vi "Register Event.vi"(4 "Get Last Broadcast Event (F)":bool, 6 "Event Handler":refnum<class "Abstract Event Message for View.lvclass">, 7 "Event":refnum<class "Event.lvclass">, 8 "error in (no error)":errorcluster, 11 "View Actor in":refnum<class "View Actor.lvclass">) -> (0 "error out":errorcluster, 3 "View Actor out":refnum<class "View Actor.lvclass">)   [LabVIEW 2023, in "Event Actors.lvlib" / "View Actor.lvclass"]
doc: "Registers an event to the Controller by specifiying the concrete event and the corresponding Event Handler."
uses:
  View Actor.lvclass
  Event Handlers/Abstract Event Message for View/Abstract Event Message for View.lvclass
  Event/Event.lvclass
  View Actor.lvclass/View Actor.ctl
  properties/Read Controller Actor Enqueuer.vi
  properties/Read Name.vi
  <vilib>/ActorFramework/Message Enqueuer/Message Enqueuer.lvclass
  Controller Actor Messages/Register by Name Msg/Register by Name Msg.lvclass
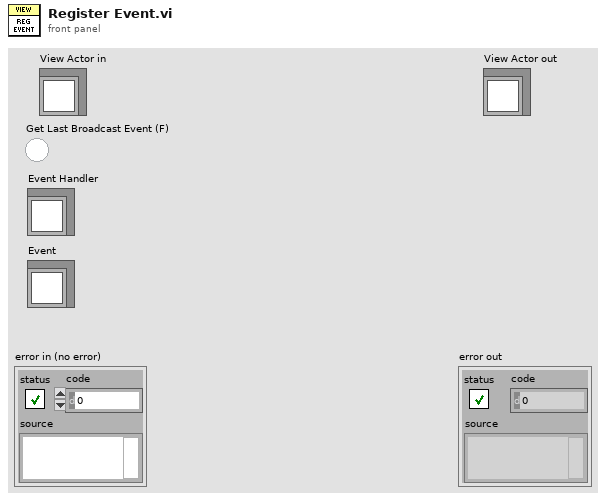
[diagram p1: front panel]
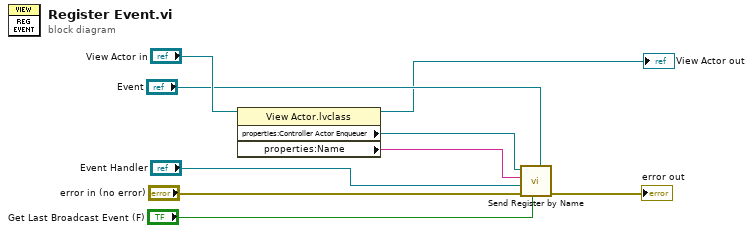
[diagram p0: block diagram]
diagram:
  n1 = property class="View Actor.lvclass"(reference="View Actor in") -> (reference out=→"View Actor out":refnum<class "View Actor.lvclass">, "properties:Controller Actor Enqueuer"=w4:refnum<class "Message Enqueuer.lvclass">, "properties:Name"=w5:string)  [unwired: 1 in, 1 out]
  n2 = call "Send Register by Name.vi"("Event"="Event", "Get Last Broadcast Event (F)"="Get Last Broadcast Event (F)", "error in (no error)"="error in (no error)", "Event Fire Handler"="Event Handler", "View Name"=w5, "Message Enqueuer in"=w4) -> ("error out"=→"error out":errorcluster)  [unwired: 4 in, 1 out]
